vi "GEvt-Convert Filter Rules - v1.0.vi"(11 "Rules-v1":T1) -> (3 "GlobalLogFilter":refnum<class "LogFilter.lvclass">)   [LabVIEW 2017, in "Communicable State Machine.lvlib"]
doc: "### GEvt-Convert Filter Rules - v1.0.vi\n\n-- <b>Controls</b> --\n- <b>Rules-v1</b>:\n\n-- <b>Indicators</b> --\n- <b>GlobalLogFilter</b>:"
uses:
  Communicable State Machine.lvlib
  LogFilter/LogFilter.lvclass
  Typedef/_CSM_GlobalLog Filter Rules - v1.0.ctl
  Typedef/_CSM_GlobalLog_MSG_TYPE.ctl
  Typedef/_CSM_GlobalLog_STATE_TYPE.ctl
  LogFilter/LogFilter.lvclass/LogFilter.ctl
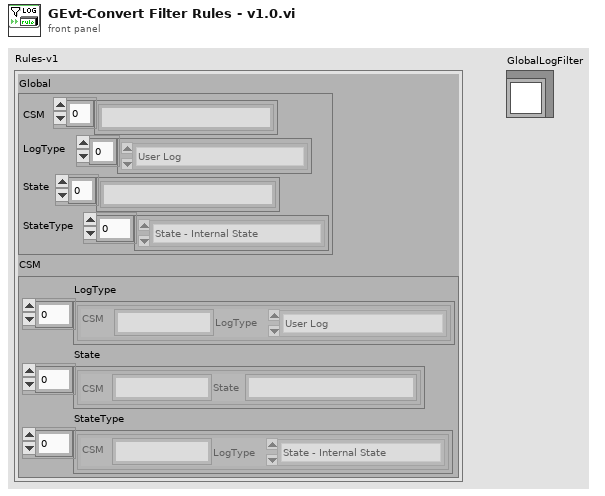
[diagram p1: front panel]
types:
  T1 = typedef "Communicable State Machine.lvlib/_CSM_GlobalLog Filter Rules - v1.0.ctl" = cluster{"Global":cluster{"CSM":string[], "LogType":T2[], "State":string[], "StateType":T3[]}, "CSM":cluster{"LogType":cluster{"CSM":string, "LogType":T2}[], "State":cluster{"CSM":string, "State":string}[], "StateType":cluster{"CSM":string, "LogType":T3}[]}}
  T2 = typedef "Communicable State Machine.lvlib/_CSM_GlobalLog_MSG_TYPE.ctl" = enum16{"User Log", "State Change", "Status", "Interrupt", "Register", "Unregister", "Error Log", "Module Created", "Module Destroyed", "Async Message", "No-Rep Async Message", "Sync Message", "AsyncMsg Complete", "SyncMsg Complete"}
  T3 = typedef "Communicable State Machine.lvlib/_CSM_GlobalLog_STATE_TYPE.ctl" = enum16{"State - Internal State", "State - External Message", "State - Response", "State - Complete"}
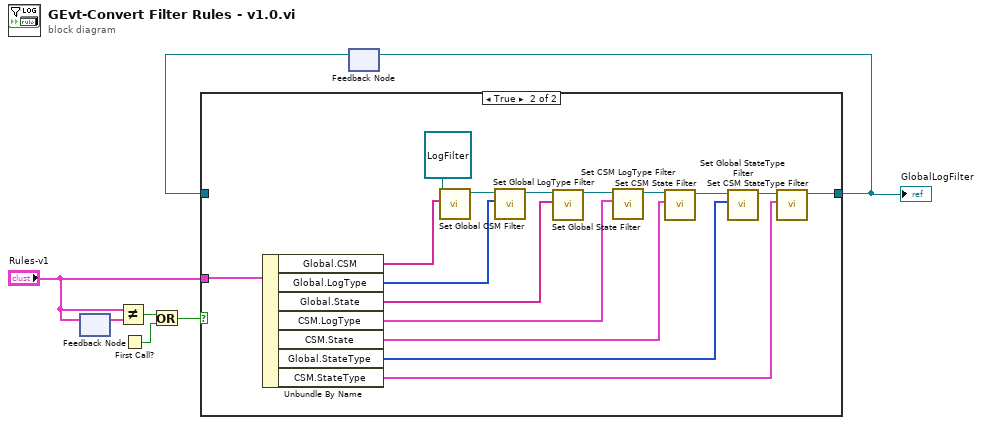
[diagram p0: block diagram]
diagram:
  n1 = feedback #1() -> (w2:T1)  [unwired: 1 in]
  n2 = feedback-in #1("Rules-v1") -> ()
  n3 = Not Equal?(x="Rules-v1", y=w2) -> (x != y?=w3:bool)
  n4 = First Call?() -> (First Call?: T/F=w4:bool)
  n5 = Or(x=w3, y=w4) -> (x .or. y?=w5:bool)
  n6 = feedback #2() -> (w7:refnum<class "LogFilter.lvclass">)  [unwired: 1 in]
  n7 = case shown="True" w5 {
    tunnel: [w8 w11] -> w6
    tunnel: "Rules-v1" -> [_ w20]
    tunnel: w7 -> [w8 _]
    frame False {
    }
    frame True {
      n8 = Unbundle By Name(w20) -> ("Global.CSM"=w22:string[], "Global.LogType"=w21:T2[], "Global.State"=w18:string[], "CSM.LogType"=w15:cluster{"CSM":string, "LogType":T2}[], "CSM.State"=w14:cluster{"CSM":string, "State":string}[], "Global.StateType"=w10:T3[], "CSM.StateType"=w9:cluster{"CSM":string, "LogType":T3}[])
      n9 = call "Set Global CSM Filter.vi"("Group:CSM"=w22, "GlobalLogFilter In"=refnum<class "LogFilter.lvclass"> refnum ("GlobalLogFilter.lvclass")) -> ("GlobalLogFilter Out"=w23:refnum<class "LogFilter.lvclass">)  [unwired: 9 in]
      n10 = call "Set Global LogType Filter.vi"("Group:LogType"=w21, "GlobalLogFilter In"=w23) -> ("GlobalLogFilter Out"=w19:refnum<class "LogFilter.lvclass">)  [unwired: 9 in]
      n11 = call "Set Global State Filter.vi"("Group:State"=w18, "GlobalLogFilter In"=w19) -> ("GlobalLogFilter Out"=w16:refnum<class "LogFilter.lvclass">)  [unwired: 9 in]
      n12 = call "Set CSM LogType Filter.vi"("LogType"=w15, "GlobalLogFilter In"=w16) -> ("GlobalLogFilter Out"=w17:refnum<class "LogFilter.lvclass">)  [unwired: 9 in]
      n13 = call "Set CSM State Filter.vi"("CSM:State"=w14, "GlobalLogFilter In"=w17) -> ("GlobalLogFilter Out"=w12:refnum<class "LogFilter.lvclass">)  [unwired: 9 in]
      n14 = call "Set Global StateType Filter.vi"("Group:LogType"=w10, "GlobalLogFilter In"=w12) -> ("GlobalLogFilter Out"=w13:refnum<class "LogFilter.lvclass">)  [unwired: 9 in]
      n15 = call "Set CSM StateType Filter.vi"("LogType"=w9, "GlobalLogFilter In"=w13) -> ("GlobalLogFilter Out"=w11:refnum<class "LogFilter.lvclass">)  [unwired: 9 in]
    }
  }
  "GlobalLogFilter" <- w6
  n16 = feedback-in #2(w6) -> ()
